vi "Write Power Mode.vi"(8 "error in (no error)":errorcluster, 10 "Power Mode":u16(ring) items=["Sleep", "Fast Measure"], 11 "H3611i Actor in":refnum<class "H3611i Actor.lvclass">) -> (0 "error out":errorcluster, 3 "H3611i Actor out":refnum<class "H3611i Actor.lvclass">)   [LabVIEW 2018, in "H3611i.lvlib" / "H3611i Actor.lvclass"]
uses:
  H3611i Actor.lvclass
  C:/Users/dev/Documents/CODE/LabVIEW/microwaveverify/trunk/MWWL Verification/Sensor Actor/Sensor/Sensor.lvclass
  H3611i Actor.lvclass/H3611i Actor.ctl
  Sensor Actor/Sensor/Sensor.lvclass
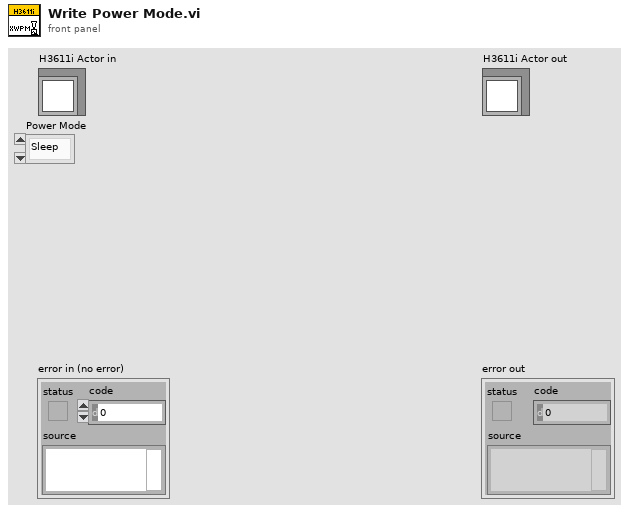
[diagram p1: front panel]
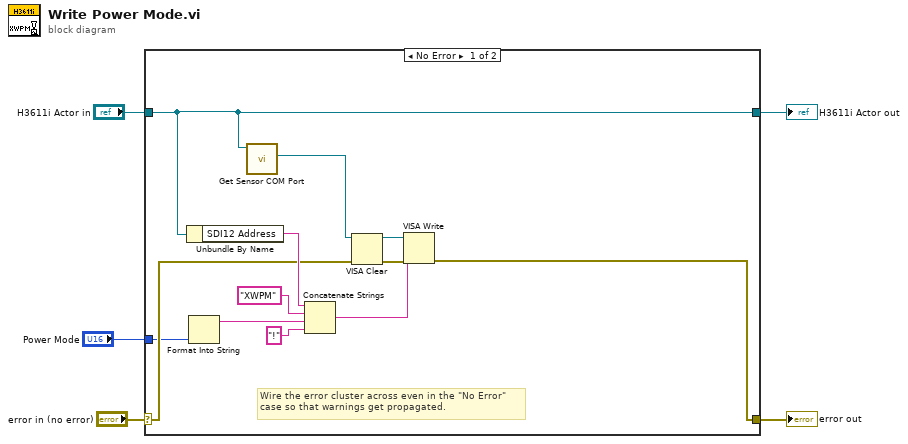
[diagram p0: block diagram]
diagram:
  n1 = case shown="No Error" "error in (no error)" {
    selector: "error in (no error)" -> [w15 w19]
    tunnel: [w8 w19] -> w4
    tunnel: [w7 w18] -> w2
    tunnel: "H3611i Actor in" -> [w7 w18]
    tunnel: "Power Mode" -> [w12 _]
    frame No Error {
      # "Wire the error cluster across even in the \"No Error\"\ncase so that warnings get propagated."
      n2 = Unbundle By Name(w7) -> ("SDI12 Address"=w17:string)
      n3 = Format Into String(w12) -> (resulting string=w10:string)  [unwired: 3 in, 1 out]
      n4 = call "Get Sensor COM Port.vi"("Sensor in"=w7) -> ("COM Port"=w6:refnum<visa-resource-name>)  [unwired: 8 in, 2 out]
      n5 = Concatenate Strings(w17, "XWPM" ("string"), w10, "!" ("string")) -> (w16:string)
      n6 = VISA Clear(VISA resource name=w6, error in (no error)=w15) -> (VISA resource name out=w13:refnum<visa-resource-name>, error out=w14:errorcluster)
      n7 = VISA Write(VISA resource name=w13, write buffer=w16, error in (no error)=w14) -> (error out=w8:errorcluster)  [unwired: 2 out]
    }
    frame Error {
    }
  }
  "error out" <- w4
  "H3611i Actor out" <- w2
